vi "MC - Create INI.vi"(4 "INI File Name":string="ballistic.ini", 5 "Fill Data":bool, 6 "Save File":bool, 7 "Key Value":string[][](array[string])=[["date&interval&message"]], 8 "Key Name":string[][](array[string])=[["reminder10"]]) -> (0 "Default OK":bool, 1 "Message Out":string[](array[string]), 2 "Interval in Days Out":string[](array[string]), 3 "Date Out":string[](array[string]), 9 "Section Name":string="Reminders(10 max)")   [LabVIEW 2015]
uses:
  Instance           4 23Saved   MC - Create INI .vi
  Instance           7 23Saved   MC - Create INI .vi
  Instance           5 23Saved   MC - Create INI .vi
  Instance           6 23Saved   MC - Create INI .vi
  Instance           9 23Saved   MC - Create INI .vi
  Instance          10 23Saved   MC - Create INI .vi
  <vilib>/Utility/config.llb/Write Key (String).vi
  <vilib>/Utility/config.llb/NI_LVConfig.lvlib
panel:
  in  "Case Constant\n(See Context Help)":bool
  in  "Exit File Bad":bool
  in  "Edit Bad Values":bool
  in  "Remove Reminder":bool
  in  "Add Reminder":bool
  in  "Exit Without Save":bool
  in  "Message":string[](array[string])
  in  "Interval in Days":string[](array[string])
  in  "Date":string[](array[string])
  in  "key control":i32 min=0
  # "Section Name"
  # "Key Name"
  # "Key Value"
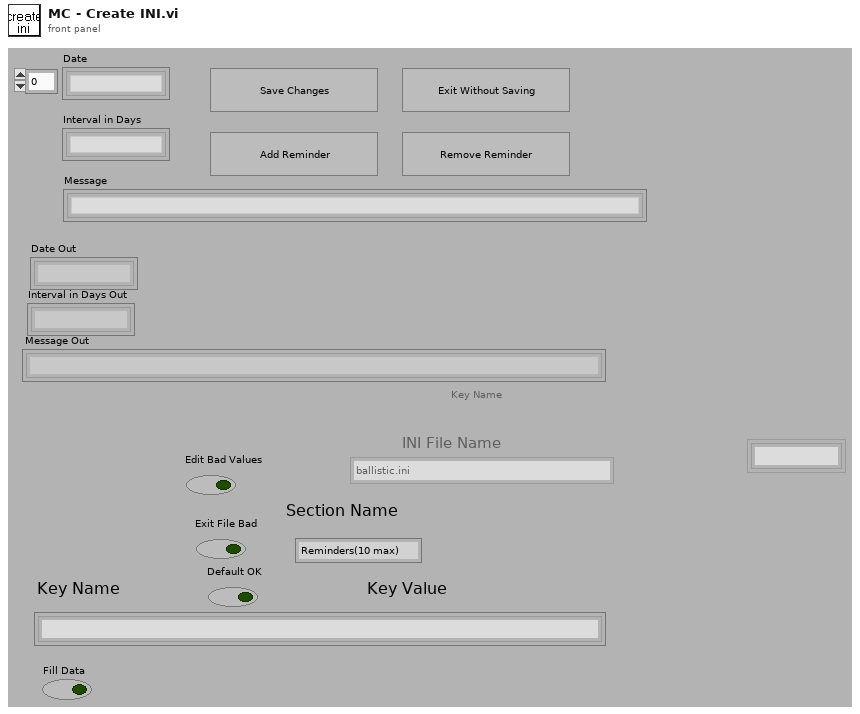
[diagram p1: front panel]
types:
  T1 = typedef "NI_LVConfig.lvlib/Config Data RefNum.ctl" = refnum<k1>
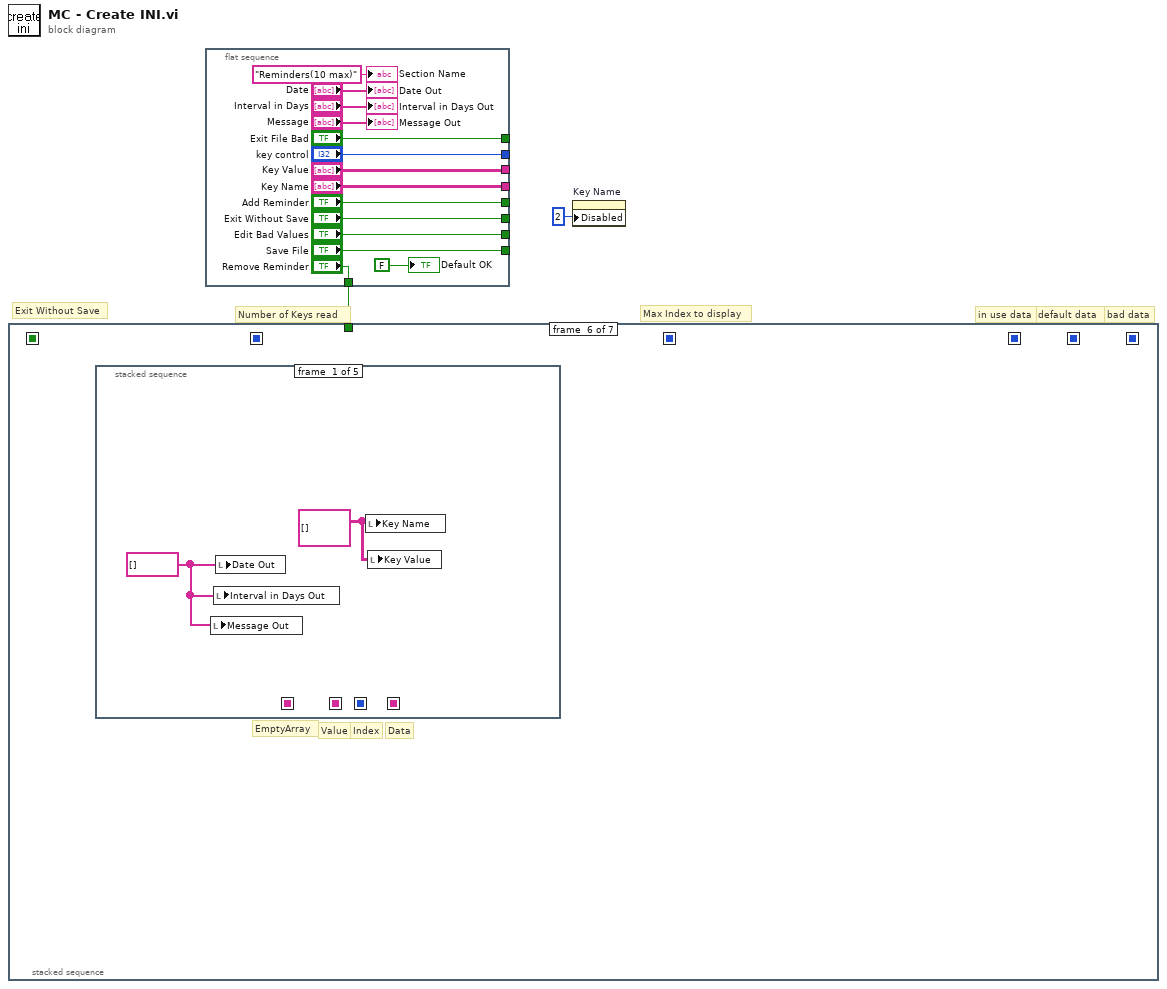
[diagram p0: block diagram]
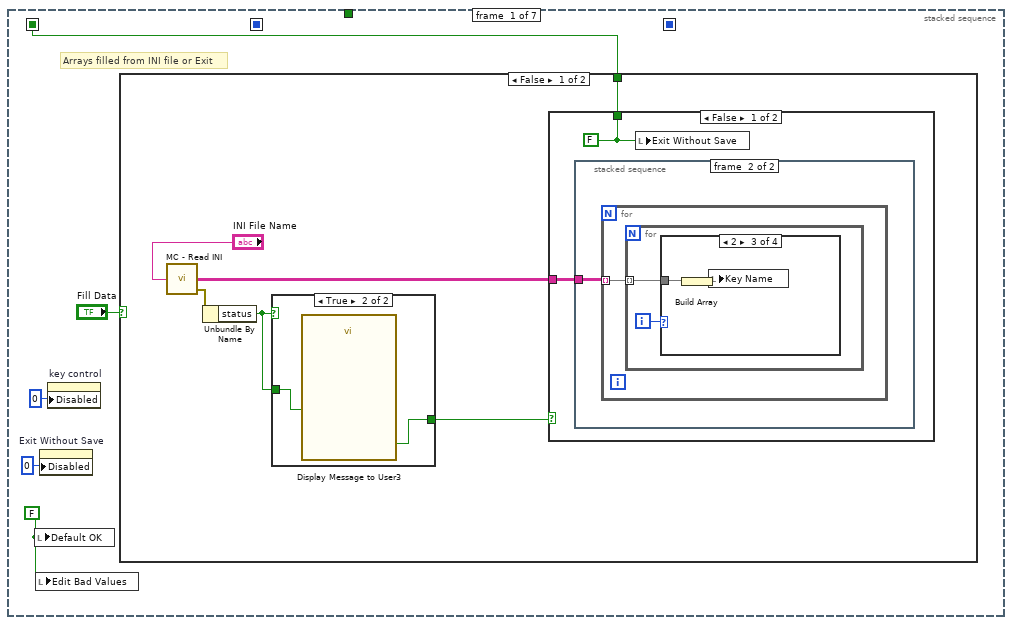
[diagram p2: hidden frame]
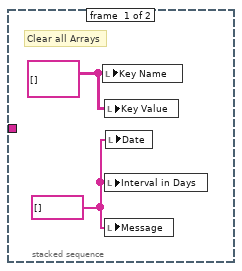
[diagram p3: hidden frame]
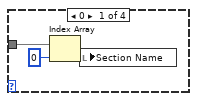
[diagram p4: hidden frame]
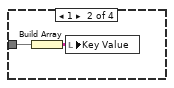
[diagram p5: hidden frame]
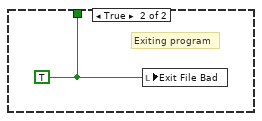
[diagram p7: hidden frame]
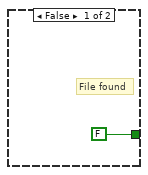
[diagram p8: hidden frame]
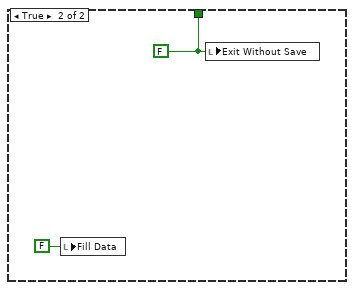
[diagram p9: hidden frame]
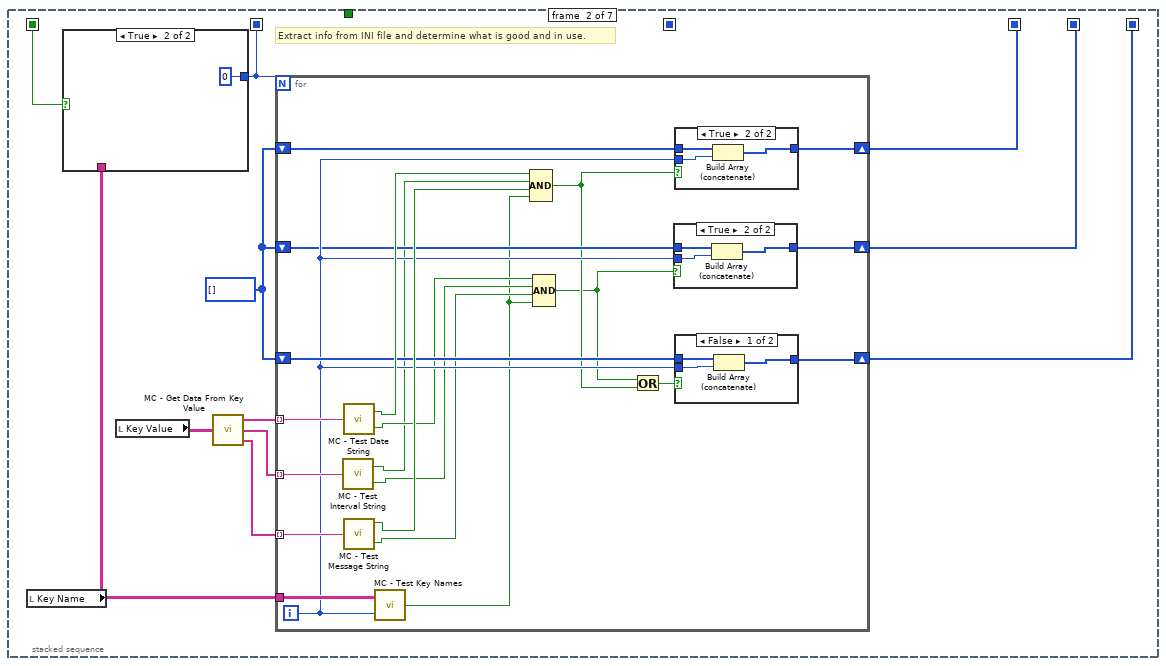
[diagram p10: hidden frame]
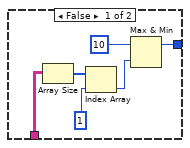
[diagram p11: hidden frame]
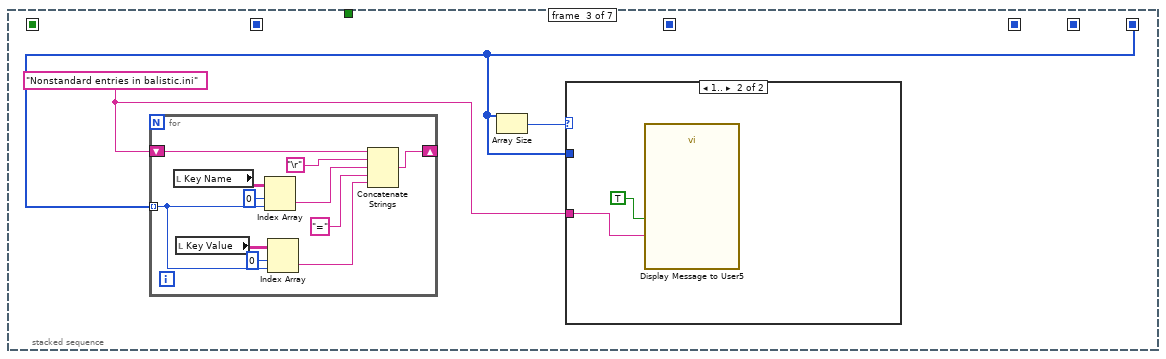
[diagram p15: hidden frame]
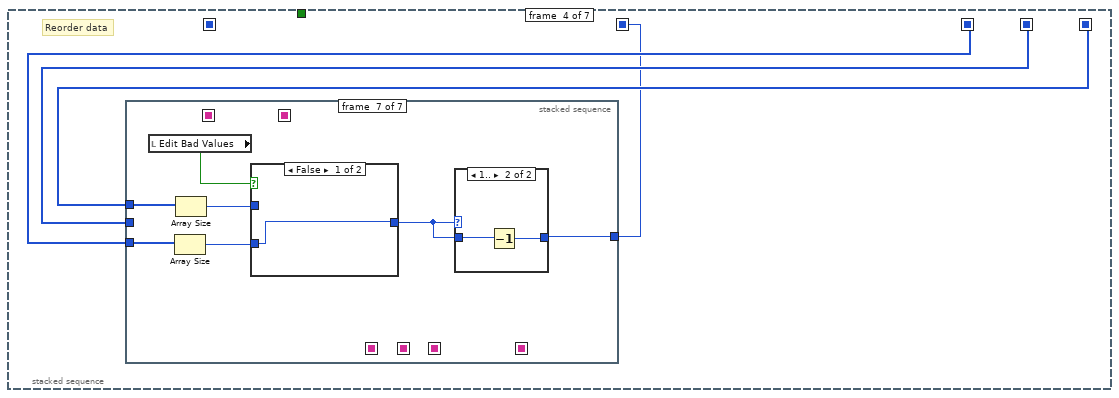
[diagram p17: hidden frame]
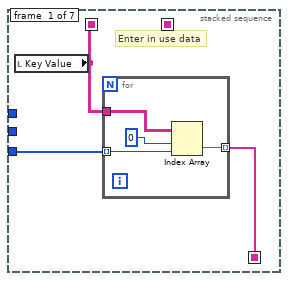
[diagram p18: hidden frame]
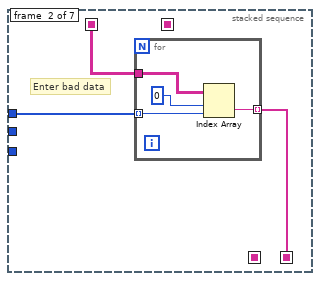
[diagram p19: hidden frame]
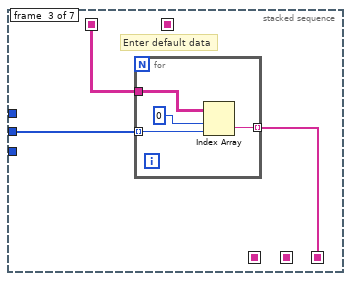
[diagram p20: hidden frame]
diagram:
  # "Max Index to display"
  # "Number of Keys read"
  # "in use data"
  # "default data"
  # "bad data"
  # "Exit Without Save"
  n1 = stacked-sequence {
    seq-local: [_ w43 _ _ _ _ _] -> [_ _ _ w103 _ _ _]
    seq-local: [w7 _ _ _ _ _ _] -> [_ w44 _ _ _ _ _]
    seq-local: [_ w42 _ _ _ _ _] -> [_ _ _ w105 _ _ _]
    seq-local: [_ w41 _ _ _ _ _] -> [_ _ _ _ _ _ _]
    seq-local: [_ w39 _ _ _ _ _] -> [_ _ w87 w104 _ _ _]
    seq-local: [_ _ _ w102 _ _ _] -> [_ _ _ _ w162 _ _]
    tunnel: w2 -> [_ _ _ _ _ _ _]
    frame #0 {
      w3 = FALSE ("Default OK")
      # "Arrays filled from INI file or Exit"
      n2 = local write "Default OK"(w3) -> ()
      n3 = local write "Edit Bad Values"(w3) -> ()
      n4 = property on="Exit Without Save" class="Bool (strict)"("Disabled"=u8 0) -> ()  [unwired: 2 in, 2 out]
      n5 = property on="key control" class="DigNum (strict)"("Disabled"=u8 0) -> ()  [unwired: 2 in, 2 out]
      n6 = case shown="False" "Fill Data" {
        tunnel: [w8 w33] -> w7
        frame False {
          n7 = call "MC - Read INI.vi"("INI Name"="INI File Name") -> ("INI Array"=w13:string[][][], "error out"=w12:errorcluster)  [unwired: 1 out]
          n8 = Unbundle By Name(w12) -> ("status"=w11:bool)
          n9 = case shown="True" w11 {
            tunnel: w11 -> [_ w32]
            tunnel: [FALSE ("OK") w31] -> w9
            frame False {
              # "File found"
            }
            frame True {
              n10 = call "Display Message to User3"("Enable"=w32) -> ("OK"=w31:bool)  [unwired: 2 in, 8 out]
            }
          }
          n11 = case shown="False" w9 {
            tunnel: w13 -> [w15 _]
            tunnel: [w14 w29] -> w8
            frame False {
              w14 = FALSE ("Exit Without Save")
              n12 = stacked-sequence {
                tunnel: w15 -> [_ w18]
                frame #0 {
                  w16 = string[] [] ("Interval in Days")
                  w17 = string[][] [] ("Array")
                  # "Clear all Arrays"
                  n13 = local write "Key Name"(w17) -> ()
                  n14 = local write "Key Value"(w17) -> ()
                  n15 = local write "Interval in Days"(w16) -> ()
                  n16 = local write "Message"(w16) -> ()
                  n17 = local write "Date"(w16) -> ()
                }
                frame #1 {
                  n18 = for {
                    tunnel: w18 -> [w19] mode=indexing
                    n19 = for {
                      tunnel: w19 -> [w20] mode=indexing
                      i -> [w21]
                      n20 = case shown="2" w21 {
                        tunnel: w20 -> [w24 w26 w28 _]
                        frame 0 {
                          n21 = Index Array(array=w24, index=0) -> (element=w22:string)
                          n22 = local write "Section Name"(w22) -> ()
                        }
                        frame 1 {
                          n23 = Build Array(w26) -> (w25:string[][])
                          n24 = local write "Key Value"(w25) -> ()
                        }
                        frame 2 {
                          n25 = Build Array(w28) -> (w27:string[][])
                          n26 = local write "Key Name"(w27) -> ()
                        }
                        frame 3, Default {
                        }
                      }
                    }
                  }
                }
              }
              n27 = local write "Exit Without Save"(w14) -> ()
            }
            frame True {
              w29 = TRUE ("Exit Without Save")
              # "Exiting program"
              n28 = local write "Exit File Bad"(w29) -> ()
            }
          }
        }
        frame True {
          w33 = FALSE ("Exit Without Save")
          n29 = local write "Fill Data"(FALSE ("Fill Data")) -> ()
          n30 = local write "Exit Without Save"(w33) -> ()
        }
      }
    }
    frame #1 {
      w40 = i32[] []
      # "Extract info from INI file and determine what is good and in use."
      n31 = local read "Key Name"() -> (w45:string[][])
      n32 = case shown="True" w44 {
        tunnel: w45 -> [w51 _]
        tunnel: [w48 0] -> w41
        frame False {
          n33 = Array Size(array=w51) -> (size(s)=w50:i32[])
          n34 = Index Array(array=w50, index=1) -> (element=w47:i32)
          n35 = Max & Min(x=10, y=w47) -> (max(x,y)=w48:i32)  [unwired: 1 out]
        }
        frame True {
        }
      }
      n36 = local read "Key Value"() -> (w38:string[][])
      n37 = call "MC - Get Data From Key Value.vi"("Key Value"=w38) -> ("Date"=w37:string[], "Interval in Days"=w36:string[], "Message"=w35:string[])
      n38 = for {
        N: w41 -> [_]
        tunnel: w45 -> [w73]
        shift-right: [w64] -> w43
        shift-left: w40 -> [w67]
        shift-right: [w62] -> w42
        shift-left: w40 -> [w61]
        shift-right: [w65] -> w39
        shift-left: w40 -> [w66]
        tunnel: w37 -> [w72] mode=indexing
        tunnel: w36 -> [w71] mode=indexing
        tunnel: w35 -> [w70] mode=indexing
        i -> [w63]
        n39 = call "MC - Test Interval String.vi"("interval string"=w71) -> ("valid interval"=w57:bool, "interval string is \"interval\""=w59:bool)
        n40 = call "MC - Test Date String.vi"("date string"=w72) -> ("valid date"=w69:bool, "the string is \"date\""=w60:bool)
        n41 = call "MC - Test Message String.vi"("message string"=w70) -> ("valid message"=w68:bool, "message string is \"message\""=w58:bool)
        n42 = call "MC - Test Key Names.vi"("index"=w63, "Key Name"=w73) -> ("key name valid"=w53:bool)
        n43 = Compound Arithmetic op=AND(w69, w57, w68, w53) -> (w55:bool)
        n44 = Compound Arithmetic op=AND(w60, w59, w58, w53) -> (w54:bool)
        n45 = Or(x=w54, y=w55) -> (x .or. y?=w56:bool)
        n46 = case shown="True" w54 {
          tunnel: w61 -> [w74 w77]
          tunnel: [w74 w76] -> w62
          tunnel: w63 -> [_ w75]
          frame False {
          }
          frame True {
            n47 = Build Array (concatenate)(w77, w75) -> (w76:i32[])
          }
        }
        n48 = case shown="True" w55 {
          tunnel: w67 -> [w82 w85]
          tunnel: [w82 w84] -> w64
          tunnel: w63 -> [_ w83]
          frame False {
          }
          frame True {
            n49 = Build Array (concatenate)(w85, w83) -> (w84:i32[])
          }
        }
        n50 = case shown="False" w56 {
          tunnel: w63 -> [w79 _]
          tunnel: w66 -> [w80 w81]
          tunnel: [w78 w81] -> w65
          frame False {
            n51 = Build Array (concatenate)(w80, w79) -> (w78:i32[])
          }
          frame True {
          }
        }
      }
    }
    frame #2 {
      w86 = "Nonstandard entries in balistic.ini"
      n52 = for {
        tunnel: w87 -> [w98] mode=indexing
        shift-right: [w91] -> _
        shift-left: w86 -> [w96]
        n53 = local read "Key Name"() -> (w101:string[][])
        n54 = local read "Key Value"() -> (w99:string[][])
        n55 = Index Array(array=w101, index (row)=0, index (col)=w98) -> (element=w94:string)
        n56 = Index Array(array=w99, index (row)=0 ("disabled index (row)"), index (col)=w98) -> (element=w92:string)
        n57 = Concatenate Strings(w96, "\r", w94, "=", w92) -> (w91:string)
      }
      n58 = Array Size(array=w87) -> (size(s)=w88:i32)
      n59 = case shown="1.." w88 {
        tunnel: w86 -> [_ w90]
        tunnel: w87 -> [_ _]
        frame ..0 {
        }
        frame 1.. {
          n60 = call "Display Message to User5"("Enable"=TRUE, "Message"=w90) -> ()  [unwired: 1 in, 9 out]
        }
      }
    }
    frame #3 {
      # "Reorder data"
      n61 = stacked-sequence {
        seq-local: [w107 _ _ _ _ _ _] -> [_ w115 w122 _ w141 _ _]
        seq-local: [w106 _ _ _ _ _ _] -> [_ _ _ w131 _ _ _]
        seq-local: [_ w113 _ _ _ _ _] -> [_ _ _ w130 _ _ _]
        seq-local: [_ _ w120 _ _ _ _] -> [_ _ _ w128 _ _ _]
        seq-local: [_ _ _ w127 _ _ _] -> [_ _ _ _ w139 _ _]
        seq-local: [_ _ _ _ w138 _ _] -> [_ _ _ _ _ w145 _]
        tunnel: w103 -> [w108 _ _ _ _ _ w150]
        tunnel: w105 -> [_ _ w121 _ _ _ _]
        tunnel: w104 -> [_ w114 _ _ _ _ w151]
        tunnel: [_ _ _ _ _ _ w146] -> w102
        frame #0 {
          # "Enter in use data"
          n62 = local read "Key Value"() -> (w107:string[][])
          n63 = for {
            tunnel: w108 -> [w110] mode=indexing
            tunnel: [w112] -> w106 mode=indexing
            tunnel: w107 -> [w111]
            n64 = Index Array(array=w111, index (row)=0 ("disabled index (col)"), index (col)=w110) -> (element=w112:string)
          }
        }
        frame #1 {
          # "Enter bad data"
          n65 = for {
            tunnel: w114 -> [w117] mode=indexing
            tunnel: [w119] -> w113 mode=indexing
            tunnel: w115 -> [w118]
            n66 = Index Array(array=w118, index (row)=0 ("disabled index (col)"), index (col)=w117) -> (element=w119:string)
          }
        }
        frame #2 {
          # "Enter default data"
          n67 = for {
            tunnel: w121 -> [w124] mode=indexing
            tunnel: [w126] -> w120 mode=indexing
            tunnel: w122 -> [w125]
            n68 = Index Array(array=w125, index (row)=0 ("disabled index (col)"), index (col)=w124) -> (element=w126:string)
          }
        }
        frame #3 {
          n69 = for {
            shift-right: [w135] -> w129
            shift-left: w131 -> [w137]
            tunnel: w130 -> [w136] mode=indexing
            n70 = Build Array (concatenate)(w137, w136) -> (w135:string[])
          }
          n71 = for {
            shift-right: [w132] -> w127
            shift-left: w129 -> [w134]
            tunnel: w128 -> [w133] mode=indexing
            n72 = Build Array (concatenate)(w134, w133) -> (w132:string[])
          }
        }
        frame #4 {
          n73 = Replace Array Subset(array=w141, new element=w139, index (row)=0) -> (w138:string[][])  [unwired: 1 in]
          n74 = local write "Key Value"(w138) -> ()
        }
        frame #5 {
          n75 = call "MC - Get Data From Key Value.vi"("Key Value"=w145) -> ("Date"=w144:string[], "Interval in Days"=w143:string[], "Message"=w142:string[])
          n76 = local write "Interval in Days"(w143) -> ()
          n77 = local write "Message"(w142) -> ()
          n78 = local write "Date"(w144) -> ()
        }
        frame #6 {
          n79 = local read "Edit Bad Values"() -> (w152:bool)
          n80 = Array Size(array=w150) -> (size(s)=w148:i32)
          n81 = Array Size(array=w151) -> (size(s)=w149:i32)
          n82 = case shown="False" w152 {
            tunnel: w149 -> [_ w159]
            tunnel: w148 -> [w156 w158]
            tunnel: [w156 w157] -> w147
            frame False {
            }
            frame True {
              n83 = Add(x=w159, y=w158) -> (x+y=w157:i32)
            }
          }
          n84 = case shown="1.." w147 {
            tunnel: [w153 w154] -> w146
            tunnel: w147 -> [w153 w155]
            frame ..0 {
            }
            frame 1.. {
              n85 = Decrement(x=w155) -> (x-1=w154:i32)
            }
          }
        }
      }
    }
    frame #4 {
      n86 = local write "key control"(0 ("key control")) -> ()
      n87 = while {
        shift-right: [w187] -> _
        shift-left: FALSE -> [w188]
        shift-right: [w186] -> _
        shift-left: FALSE -> [w185]
        shift-right: [w182] -> _
        shift-left: FALSE -> [w184]
        shift-right: [w181] -> _
        shift-left: FALSE -> [w183]
        shift-right: [w178] -> _
        shift-left: FALSE -> [w180]
        shift-right: [w177] -> _
        shift-left: FALSE -> [w179]
        shift-right: [w175] -> _
        shift-left: w162 -> [w176]
        shift-right: [w173] -> _
        shift-left: FALSE -> [w174]
        shift-right: [w170] -> _
        shift-left: -1 -> [w171]
        stop <- w172 stop-if-true
        # "Max Index Range"
        # "Default"
        # "message"
        # "interval"
        # "date"
        n88 = stacked-sequence {
          seq-local: [w191 _ _ _ _ _ _ _ _] -> [_ w211 _ _ _ w315 _ w333 _]
          seq-local: [_ w205 _ _ _ _ _ _ _] -> [_ _ _ _ w274 w314 _ _ _]
          seq-local: [_ w204 _ _ _ _ _ _ _] -> [_ _ _ w245 _ w313 _ _ _]
          seq-local: [_ w202 _ _ _ _ _ _ _] -> [_ _ w216 _ _ w312 _ _ _]
          seq-local: [_ w197 _ _ _ _ _ _ _] -> [_ _ w215 w244 w273 w309 w325 _ _]
          seq-local: [_ _ _ _ _ w305 _ _ _] -> [_ _ _ _ _ _ _ w332 _]
          tunnel: w188 -> [_ _ w223 w248 w277 _ _ _ _]
          tunnel: [_ _ w221 _ _ _ _ _ _] -> w187
          tunnel: [_ _ w220 _ _ _ _ _ _] -> w186
          tunnel: w185 -> [_ _ w222 _ _ _ _ _ _]
          tunnel: w184 -> [_ _ w219 w252 w276 _ _ _ _]
          tunnel: w183 -> [_ _ _ w251 _ _ _ _ _]
          tunnel: [_ _ _ w249 _ _ _ _ _] -> w182
          tunnel: [_ _ _ w250 _ _ _ _ _] -> w181
          tunnel: w180 -> [_ _ w218 w247 w281 _ _ _ _]
          tunnel: w179 -> [_ _ _ _ w280 _ _ _ _]
          tunnel: [_ _ _ _ w279 _ _ _ _] -> w178
          tunnel: [_ _ _ _ w278 _ _ _ _] -> w177
          tunnel: w176 -> [w190 _ _ _ _ w304 _ _ w364]
          tunnel: [_ _ _ _ _ _ _ w331 _] -> w175
          tunnel: w174 -> [_ _ _ _ _ _ w324 _ _]
          tunnel: [_ _ _ _ _ _ w323 _ _] -> w173
          tunnel: [_ _ _ _ _ _ _ _ w369] -> w172
          tunnel: w171 -> [_ _ _ _ _ _ _ _ w366]
          tunnel: [_ _ _ _ _ _ _ _ w365] -> w170
          frame #0 {
            # "Make all arrays index same value"
            n89 = local read "key control"() -> (w189:i32)
            n90 = Max & Min(x=w189, y=w190) -> (min(x,y)=w191:i32)  [unwired: 1 out]
            n91 = Build Array(0 ("Index"), w191) -> (w194:i32[])
            n92 = Build Array(w191) -> (w192:i32[])
            n93 = property on="Key Value" class="Arr (strict)"("Index Values"=w194) -> ()  [unwired: 2 in, 2 out]
            n94 = property on="Date" class="Arr (strict)"("Index Values"=w192) -> ()  [unwired: 2 in, 2 out]
            n95 = property on="Key Name" class="Arr (strict)"("Index Values"=w194) -> ()  [unwired: 2 in, 2 out]
            n96 = property on="Message" class="Arr (strict)"("Index Values"=w192) -> ()  [unwired: 2 in, 2 out]
            n97 = property on="Interval in Days" class="Arr (strict)"("Index Values"=w192) -> ()  [unwired: 2 in, 2 out]
            n98 = case shown="..9" w191 {
              tunnel: w191 -> [w195 _]
              frame ..9 {
                n99 = local write "key control"(w195) -> ()
              }
              frame 10.. {
                n100 = local write "key control"(0 ("key control")) -> ()
              }
            }
          }
          frame #1 {
            n101 = local read "Interval in Days"() -> (w213:string[])
            n102 = local read "Message"() -> (w212:string[])
            n103 = local read "Date"() -> (w214:string[])
            n104 = Index Array(array=w214, index=w211) -> (element=w208:string)
            n105 = Index Array(array=w213, index=w211) -> (element=w209:string)
            n106 = Index Array(array=w212, index=w211) -> (element=w210:string)
            n107 = call "MC - Test Date String.vi"("date string"=w208) -> ("valid date"=w203:bool, "the string is \"date\""=w201:bool)
            n108 = call "MC - Test Interval String.vi"("interval string"=w209) -> ("valid interval"=w207:bool, "interval string is \"interval\""=w200:bool)
            n109 = call "MC - Test Message String.vi"("message string"=w210) -> ("valid message"=w206:bool, "message string is \"message\""=w199:bool)
            n110 = Not(x=w203) -> (.not. x?=w202:bool)
            n111 = Not(x=w207) -> (.not. x?=w204:bool)
            n112 = Not(x=w206) -> (.not. x?=w205:bool)
            n113 = Compound Arithmetic op=AND(w201, w200, w199) -> (w198:bool)
            n114 = Not(x=w198) -> (.not. x?=w197:bool)
          }
          frame #2 {
            n115 = And(x=w216, y=w215) -> (x .and. y?=w217:bool)
            n116 = case shown="True" w217 {
              tunnel: w223 -> [w227 w237]
              tunnel: w222 -> [w229 w236]
              tunnel: [FALSE w235] -> w221
              tunnel: [w229 w234] -> w220
              tunnel: w219 -> [w226 _]
              tunnel: w218 -> [w225 _]
              frame False {
                n117 = Or(x=w226, y=w225) -> (x .or. y?=w224:bool)
                n118 = case shown="True" w227 {
                  tunnel: w224 -> [_ w230]
                  frame False {
                  }
                  frame True {
                    n119 = case shown="False" w230 {
                      frame False {
                        w231 = u8 0 ("Disabled")
                        n120 = property on="key control" class="DigNum (strict)"("Disabled"=w231) -> ()  [unwired: 2 in, 2 out]
                        n121 = property on="Save File" class="Bool (strict)"("Disabled"=w231) -> ()  [unwired: 2 in, 2 out]
                      }
                      frame True {
                      }
                    }
                  }
                }
              }
              frame True {
                n122 = call "Display Message to User4"("Enable"=w236) -> ("OK"=w238:bool)  [unwired: 2 in, 8 out]
                n123 = Or(x=w237, y=w238) -> (x .or. y?=w233:bool)
                n124 = case shown="False" w233 {
                  tunnel: [FALSE TRUE] -> w235
                  tunnel: [TRUE FALSE] -> w234
                  frame False {
                    w239 = u8 2 ("Disabled")
                    n125 = property on="key control" class="DigNum (strict)"("Disabled"=w239) -> ()  [unwired: 2 in, 2 out]
                    n126 = property on="Add Reminder" class="Bool (strict)"("Disabled"=w239) -> ()  [unwired: 2 in, 2 out]
                    n127 = property on="Save File" class="Bool (strict)"("Disabled"=w239) -> ()  [unwired: 2 in, 2 out]
                  }
                  frame True {
                  }
                }
                n128 = local write "Save File"(FALSE ("Save File")) -> ()
              }
            }
          }
          frame #3 {
            n129 = And(x=w245, y=w244) -> (x .and. y?=w246:bool)
            n130 = case shown="True" w246 {
              tunnel: w252 -> [w253 w267]
              tunnel: w251 -> [w258 w266]
              tunnel: [FALSE w264] -> w249
              tunnel: [w258 w263] -> w250
              tunnel: w248 -> [w257 _]
              tunnel: w247 -> [w256 _]
              frame False {
                n131 = Or(x=w257, y=w256) -> (x .or. y?=w254:bool)
                n132 = case shown="True" w253 {
                  tunnel: w254 -> [_ w259]
                  frame False {
                  }
                  frame True {
                    n133 = case shown="False" w259 {
                      frame False {
                        w260 = u8 0 ("Disabled")
                        n134 = property on="key control" class="DigNum (strict)"("Disabled"=w260) -> ()  [unwired: 2 in, 2 out]
                        n135 = property on="Save File" class="Bool (strict)"("Disabled"=w260) -> ()  [unwired: 2 in, 2 out]
                      }
                      frame True {
                      }
                    }
                  }
                }
              }
              frame True {
                n136 = call "Display Message to User"("Enable"=w266) -> ("OK"=w265:bool)  [unwired: 2 in, 8 out]
                n137 = Or(x=w267, y=w265) -> (x .or. y?=w262:bool)
                n138 = case shown="False" w262 {
                  tunnel: [FALSE TRUE] -> w264
                  tunnel: [TRUE FALSE] -> w263
                  frame False {
                    w268 = u8 2 ("Disabled")
                    n139 = property on="key control" class="DigNum (strict)"("Disabled"=w268) -> ()  [unwired: 2 in, 2 out]
                    n140 = property on="Add Reminder" class="Bool (strict)"("Disabled"=w268) -> ()  [unwired: 2 in, 2 out]
                    n141 = property on="Save File" class="Bool (strict)"("Disabled"=w268) -> ()  [unwired: 2 in, 2 out]
                  }
                  frame True {
                  }
                }
                n142 = local write "Save File"(FALSE ("Save File")) -> ()
              }
            }
          }
          frame #4 {
            n143 = And(x=w274, y=w273) -> (x .and. y?=w275:bool)
            n144 = case shown="True" w275 {
              tunnel: [FALSE w294] -> w279
              tunnel: [w287 w293] -> w278
              tunnel: w281 -> [w283 w291]
              tunnel: w280 -> [w287 w292]
              tunnel: w277 -> [w285 _]
              tunnel: w276 -> [w284 _]
              frame False {
                n145 = Or(x=w285, y=w284) -> (x .or. y?=w282:bool)
                n146 = case shown="True" w283 {
                  tunnel: w282 -> [_ w288]
                  frame False {
                  }
                  frame True {
                    n147 = case shown="False" w288 {
                      frame False {
                        w289 = u8 0 ("Disabled")
                        n148 = property on="key control" class="DigNum (strict)"("Disabled"=w289) -> ()  [unwired: 2 in, 2 out]
                        n149 = property on="Save File" class="Bool (strict)"("Disabled"=w289) -> ()  [unwired: 2 in, 2 out]
                      }
                      frame True {
                      }
                    }
                  }
                }
              }
              frame True {
                n150 = call "Display Message to User7"("Enable"=w292) -> ("OK"=w296:bool)  [unwired: 2 in, 8 out]
                n151 = Or(x=w291, y=w296) -> (x .or. y?=w295:bool)
                n152 = case shown="False" w295 {
                  tunnel: [FALSE TRUE] -> w294
                  tunnel: [TRUE FALSE] -> w293
                  frame False {
                    w297 = u8 2 ("Disabled")
                    n153 = property on="key control" class="DigNum (strict)"("Disabled"=w297) -> ()  [unwired: 2 in, 2 out]
                    n154 = property on="Add Reminder" class="Bool (strict)"("Disabled"=w297) -> ()  [unwired: 2 in, 2 out]
                    n155 = property on="Save File" class="Bool (strict)"("Disabled"=w297) -> ()  [unwired: 2 in, 2 out]
                  }
                  frame True {
                  }
                }
                n156 = local write "Save File"(FALSE ("Save File")) -> ()
              }
            }
          }
          frame #5 {
            n157 = Equal?(x=w304, y=w315) -> (x = y?=w307:bool)
            n158 = Not(x=w307) -> (.not. x?=w306:bool)
            n159 = Equal?(x=w304, y=9) -> (x = y?=w302:bool)
            n160 = Not(x=w309) -> (.not. x?=w310:bool)
            n161 = Compound Arithmetic op=OR(w302, w306, w314, w313, w312, w310) -> (w308:bool)
            n162 = case shown="False" w308 {
              tunnel: [0 2] -> w311
              frame False {
              }
              frame True {
              }
            }
            n163 = local read "Add Reminder"() -> (w316:bool)
            n164 = property on="Add Reminder" class="Bool (strict)"("Disabled"=w311) -> ()  [unwired: 2 in, 2 out]
            n165 = case shown="True" w316 {
              tunnel: w304 -> [w319 w322]
              tunnel: [w319 w320] -> w305
              frame False {
              }
              frame True {
                n166 = Increment(x=w322) -> (x+1=w320:i32)
                n167 = local write "Add Reminder"(FALSE) -> ()
                n168 = local write "key control"(w320) -> ()
              }
            }
          }
          frame #6 {
            n169 = case shown="False" w325 {
              tunnel: w324 -> [w327 _]
              tunnel: [FALSE TRUE] -> w323
              frame False {
                n170 = case shown="True" w327 {
                  frame False {
                  }
                  frame True {
                    w328 = u8 0 ("Disabled")
                    n171 = property on="key control" class="DigNum (strict)"("Disabled"=w328) -> ()  [unwired: 2 in, 2 out]
                    n172 = property on="Save File" class="Bool (strict)"("Disabled"=w328) -> ()  [unwired: 2 in, 2 out]
                  }
                }
              }
              frame True {
              }
            }
          }
          frame #7 {
            n173 = local read "Remove Reminder"() -> (w330:bool)
            n174 = case shown="True" w330 {
              tunnel: w333 -> [_ w338]
              tunnel: w332 -> [w334 w337]
              tunnel: [w334 w336] -> w331
              frame False {
              }
              frame True {
                n175 = stacked-sequence {
                  seq-local: [w339 _] -> [_ w343]
                  tunnel: w338 -> [_ w344]
                  tunnel: w337 -> [_ w342]
                  tunnel: [_ w341] -> w336
                  frame #0 {
                    n176 = call "Display Message to User2"("Enable"=TRUE) -> ("OK"=w339:bool)  [unwired: 2 in, 8 out]
                  }
                  frame #1 {
                    n177 = case shown="True" w343 {
                      tunnel: w344 -> [_ w348]
                      tunnel: w342 -> [w345 w347]
                      tunnel: [w345 w346] -> w341
                      frame False {
                      }
                      frame True {
                        n178 = stacked-sequence {
                          tunnel: w348 -> [w352 _ _]
                          tunnel: w347 -> [_ w356 _]
                          tunnel: [_ w357 _] -> w346
                          frame #0 {
                            n179 = local read "Interval in Days"() -> (w354:string[])
                            n180 = local read "Message"() -> (w353:string[])
                            n181 = local read "Date"() -> (w355:string[])
                            n182 = Delete From Array(array=w355, index=w352) -> (array with subset deleted=w351:string[])  [unwired: 1 in, 1 out]
                            n183 = Delete From Array(array=w354, index=w352) -> (array with subset deleted=w350:string[])  [unwired: 1 in, 1 out]
                            n184 = Delete From Array(array=w353, index=w352) -> (array with subset deleted=w349:string[])  [unwired: 1 in, 1 out]
                            n185 = local write "Message"(w349) -> ()
                            n186 = local write "Interval in Days"(w350) -> ()
                            n187 = local write "Date"(w351) -> ()
                          }
                          frame #1 {
                            n188 = case shown="..0" w356 {
                              tunnel: w356 -> [w358 w360]
                              tunnel: [w358 w359] -> w357
                              frame ..0 {
                              }
                              frame 1.. {
                                n189 = Decrement(x=w360) -> (x-1=w359:i32)
                              }
                            }
                          }
                          frame #2 {
                            n190 = property on="Save File" class="Bool (strict)"("Disabled"=u8 0) -> ()  [unwired: 2 in, 2 out]
                          }
                        }
                      }
                    }
                  }
                }
                n191 = local write "Remove Reminder"(FALSE ("Remove Reminder")) -> ()
              }
            }
          }
          frame #8 {
            n192 = local read "Save File"() -> (w367:bool)
            n193 = case shown="True" w367 {
              tunnel: w366 -> [w371 w374]
              tunnel: [w371 w375] -> w365
              tunnel: w364 -> [_ w373]
              tunnel: [FALSE w372] -> w363
              frame False {
              }
              frame True {
                n194 = Equal?(x=w373, y=w374) -> (x = y?=w372:bool)
                n195 = Increment(x=w374) -> (x+1=w375:i32)
                n196 = local write "key control"(w375) -> ()
              }
            }
            n197 = local read "Exit Without Save"() -> (w368:bool)
            n198 = local read "Exit File Bad"() -> (w362:bool)
            n199 = Compound Arithmetic op=OR(w363, w368, w362) -> (w369:bool)
          }
        }
      }
    }
    frame #5 {
      # "Data"
      # "Index"
      # "Value"
      # "EmptyArray"
      n200 = stacked-sequence {
        seq-local: [_ w378 _ _ _] -> [_ _ w383 _ _]
        seq-local: [_ _ w382 _ _] -> [_ _ _ _ w400]
        seq-local: [_ _ _ w390 _] -> [_ _ _ _ _]
        seq-local: [_ _ _ w389 _] -> [_ _ _ _ w398]
        frame #0 {
          w376 = string[] []
          w377 = string[][] []
          n201 = local write "Message Out"(w376) -> ()
          n202 = local write "Interval in Days Out"(w376) -> ()
          n203 = local write "Date Out"(w376) -> ()
          n204 = local write "Key Name"(w377) -> ()
          n205 = local write "Key Value"(w377) -> ()
        }
        frame #1 {
          n206 = Initialize Array("", 1 ("dimension size"), 10 ("dimension size")) -> (w378:string[][])
        }
        frame #2 {
          n207 = call "MC - Fill Default Values.vi"("Key Value In"=w383, "Key Name In"=w383, "Array of Bad Data"=i32[] [0, 1, 2, 3, 4, 5, 6, 7, 8, 9]) -> ("Key Value Out"=w382:string[][], "Key Name Out"=w385:string[][])
          n208 = local write "Key Value"(w382) -> ()
          n209 = local write "Key Name"(w385) -> ()
        }
        frame #3 {
          n210 = local read "Interval in Days"() -> (w387:string[])
          n211 = local read "Message"() -> (w388:string[])
          n212 = local read "Date"() -> (w386:string[])
          n213 = local write "Interval in Days Out"(w387) -> ()
          n214 = local write "Message Out"(w388) -> ()
          n215 = local write "Date Out"(w386) -> ()
          n216 = for {
            tunnel: w386 -> [w396] mode=indexing
            tunnel: w387 -> [w394] mode=indexing
            tunnel: w388 -> [w393] mode=indexing
            tunnel: [w392] -> w389 mode=indexing
            tunnel: [w391] -> w390
            i -> [w391]
            w395 = "&"
            n217 = Concatenate Strings(w396, w395, w394, w395, w393) -> (w392:string)
          }
        }
        frame #4 {
          n218 = Replace Array Subset(array=w400, new element=w398, index (row)=0) -> (w397:string[][])  [unwired: 1 in]
          n219 = local write "Key Value"(w397) -> ()
        }
      }
    }
    frame #6 {
      w401 = FALSE ("Save File")
      n220 = local read "Exit Without Save"() -> (w402:bool)
      n221 = case shown="False" w402 {
        frame False {
          n222 = stacked-sequence {
            seq-local: [w409 _] -> [_ w450]
            seq-local: [w408 _] -> [_ w451]
            frame #0 {
              w416 = FALSE  # create file if necessary? (T)
              n223 = case shown="True" "Case Constant\n(See Context Help)" {
                frame False {
                }
                frame True {
                  n224 = Current VI's Path() -> (path=w418:path)
                  n225 = for {
                    N: 2 -> [_]
                    shift-right: [w421] -> w419
                    shift-left: w418 -> [w422]
                    n226 = File/Directory Info(path=w422) -> (directory=w423:bool)  [unwired: 1 in, 6 out]
                    n227 = case shown="True" w423 {
                      tunnel: w422 -> [w425 w426]
                      tunnel: [w424 w426] -> w421
                      frame False {
                        n228 = Strip Path(path=w425) -> (stripped path=w424:path)  [unwired: 1 out]
                      }
                      frame True {
                      }
                    }
                  }
                  n229 = local read "INI File Name"() -> (w417:string)
                  n230 = Build Path(base path=w419, name or relative path=w417) -> ()  [unwired: 1 out]
                }
              }
              n231 = local read "INI File Name"() -> (w404:string)
              n232 = local read "Section Name"() -> (w412:string)
              n233 = String To Path(string=w404) -> (path=w403:path)
              n234 = call <vilib>:"Open Config Data (compatibility).vi"("create file if necessary (T)"=w416, "configuration file path"=w403) -> ("error out"=w410:errorcluster, "refnum"=w411:T1)  [unwired: 7 in, 1 out]
              n235 = call <vilib>:"Get Key Names.vi"("section"=w412, "error in (no error)"=w410, "refnum"=w411) -> ("error out"=w414:errorcluster, "key names"=w406:string[], "section exists?"=w413:bool, "refnum out"=w415:T1)  [unwired: 5 out]
              n236 = Array Size(array=w406) -> (size(s)=w407:i32)
              n237 = case shown="..0" w407 {
                tunnel: w415 -> [w428 w435]
                tunnel: w414 -> [w427 w434]
                tunnel: w413 -> [_ w433]
                tunnel: w412 -> [_ w432]
                tunnel: [w427 w431] -> w409
                tunnel: [w428 w430] -> w408
                tunnel: w406 -> [_ w429]
                frame ..0 {
                }
                frame 1.. {
                  n238 = case shown="False" w433 {
                    tunnel: w429 -> [_ w443]
                    tunnel: w435 -> [w437 w442]
                    tunnel: w434 -> [w436 w441]
                    tunnel: [w437 w440] -> w430
                    tunnel: [w436 w439] -> w431
                    tunnel: w432 -> [_ w438]
                    frame False {
                    }
                    frame True {
                      n239 = for {
                        tunnel: w443 -> [w448] mode=indexing
                        tunnel: w442 -> [w449]
                        tunnel: w441 -> [w447]
                        tunnel: [w446] -> w440
                        tunnel: [w445] -> w439
                        tunnel: w438 -> [w444]
                        n240 = call <vilib>:"Remove Key.vi"("section"=w444, "error in (no error)"=w447, "key"=w448, "refnum"=w449) -> ("error out"=w445:errorcluster, "refnum out"=w446:T1)  [unwired: 6 out]
                      }
                    }
                  }
                }
              }
            }
            frame #1 {
              n241 = local read "Section Name"() -> (w457:string)
              n242 = local read "Key Name"() -> (w453:string[][])
              n243 = local read "Key Value"() -> (w452:string[][])
              n244 = for {
                N: 1 -> [_]
                tunnel: w457 -> [w459]
                tunnel: w451 -> [w468]
                tunnel: [w467] -> w454
                tunnel: [w466] -> w455
                tunnel: w450 -> [w462]
                tunnel: w453 -> [w461]
                tunnel: w452 -> [w460]
                i -> [w464]
                n245 = Index Array(array=w461, index (row)=w464) -> (element=w465:string[])  [unwired: 1 in]
                n246 = Index Array(array=w460, index (row)=w464) -> (element=w463:string[])  [unwired: 1 in]
                n247 = Array Size(array=w465) -> (size(s)=w469:i32)
                n248 = for {
                  N: w469 -> [_]
                  tunnel: w465 -> [w479]
                  tunnel: w463 -> [w480]
                  tunnel: w459 -> [w477]
                  tunnel: w468 -> [w481]
                  tunnel: [w476] -> w467
                  tunnel: [w475] -> w466
                  tunnel: w462 -> [w470]
                  i -> [w474]
                  n249 = Index Array(array=w479, index=w474) -> (element=w473:string)
                  n250 = Index Array(array=w480, index=w474) -> (element=w478:string)
                  n251 = Equal?(x=w473, y="") -> (x = y?=w471:bool)
                  n252 = case shown="False" w471 {
                    tunnel: w481 -> [w488 w490]
                    tunnel: w473 -> [w487 _]
                    tunnel: w478 -> [w486 _]
                    tunnel: w477 -> [w485 _]
                    tunnel: [w484 w490] -> w476
                    tunnel: [w483 w489] -> w475
                    tunnel: w470 -> [w482 w489]
                    frame False {
                      n253 = call-poly <vilib>:"Write Key.vi"("section"=w485, "error in (no error)"=w482, "value"=w486, "key"=w487, "refnum"=w488) -> ("error out"=w483:errorcluster, "refnum out"=w484:T1)  [unwired: 1 in, 4 out]
                    }
                    frame True {
                    }
                  }
                }
              }
              n254 = call <vilib>:"Close Config Data.vi"("error in (no error)"=w455, "write file if changed (T)"=TRUE ("write configuration file? (F)"), "refnum"=w454) -> ()  [unwired: 9 out]
            }
          }
        }
        frame True {
          n255 = local read "Key Value"() -> (w491:string[][])
          n256 = call "MC - Get Data From Key Value.vi"("Key Value"=w491) -> ("Date"=w494:string[], "Interval in Days"=w493:string[], "Message"=w492:string[])
          n257 = local write "Interval in Days"(w493) -> ()
          n258 = local write "Message"(w492) -> ()
          n259 = local write "Date"(w494) -> ()
          n260 = local write "Exit Without Save"(FALSE ("Exit Without Save")) -> ()
        }
      }
      n261 = local write "Save File"(w401) -> ()
      n262 = local write "Exit File Bad"(w401) -> ()
    }
  }
  n263 = flat-sequence {
    tunnel: ["Remove Reminder"] -> w2
    tunnel: ["Exit File Bad"] -> _
    tunnel: ["key control"] -> _
    tunnel: ["Key Value"] -> _
    tunnel: ["Key Name"] -> _
    tunnel: ["Add Reminder"] -> _
    tunnel: ["Exit Without Save"] -> _
    tunnel: ["Edit Bad Values"] -> _
    tunnel: ["Save File"] -> _
    frame #0 {
      "Section Name" <- "Reminders(10 max)" ("Section Name")
      "Message Out" <- "Message"
      "Date Out" <- "Date"
      "Interval in Days Out" <- "Interval in Days"
      "Default OK" <- FALSE ("Default OK")
    }
  }
  n264 = property on="Key Name" class="Arr (strict)"("Disabled"=u8 2) -> ()  [unwired: 2 in, 2 out]
